vi "fittedresultdisplay.vi"(9 "x":dbl[](array[numeric]), 10 "num of gaussian peaks":i32, 11 "best fit parameters":dbl[](array[numeric])) -> (2 "resulting formula string":string, 3 "all gaussian points":T1(array[cluster]))   [LabVIEW 2020]
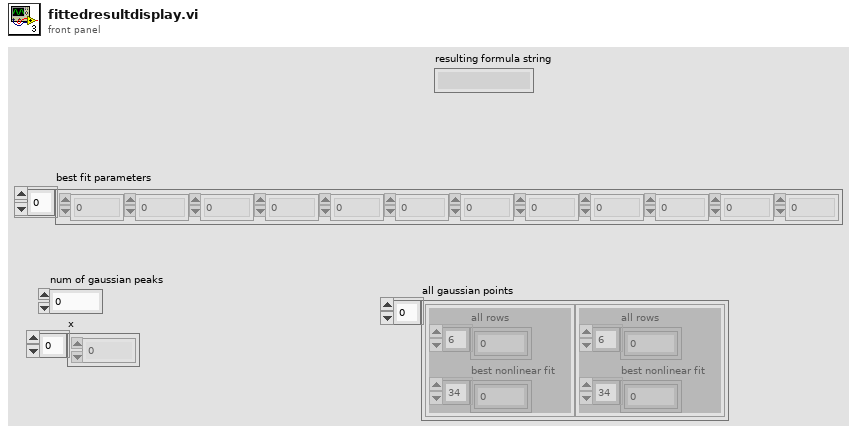
[diagram p1: front panel]
types:
  T1 = cluster{"all rows":dbl[], "best nonlinear fit":dbl[]}[]
  T2 = cluster{"all rows":dbl[], "best nonlinear fit":dbl[]}
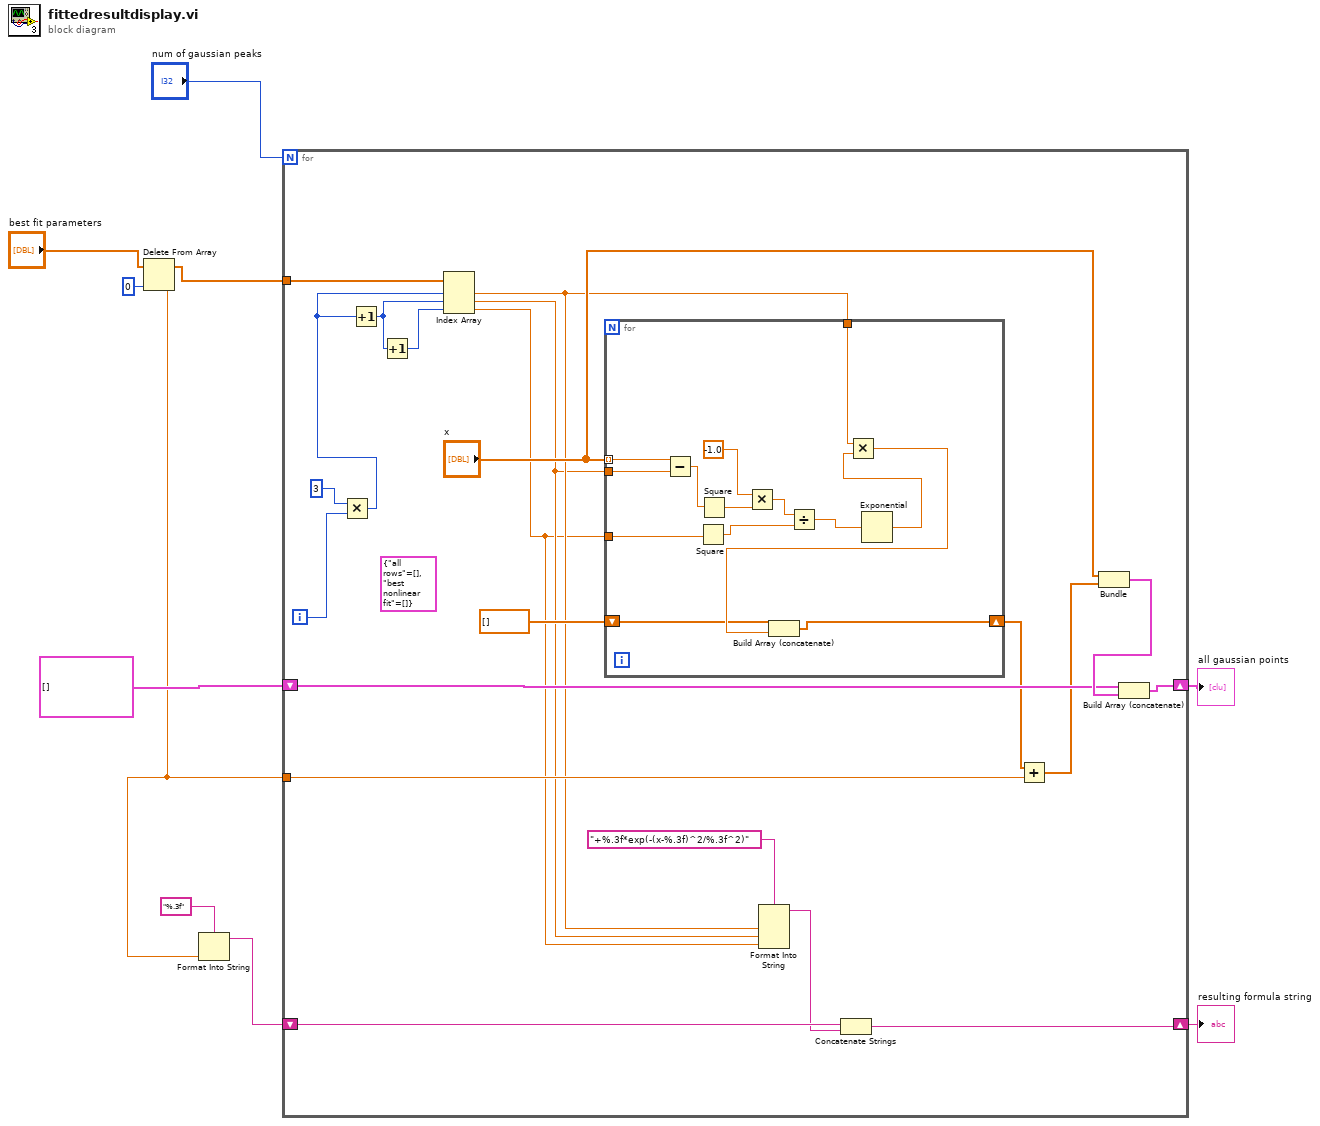
[diagram p0: block diagram]
diagram:
  n1 = Delete From Array(array="best fit parameters", index=0) -> (deleted portion=w3:dbl, array with subset deleted=w5:dbl[])  [unwired: 1 in]
  n2 = Format Into String(format string="%.3f", w3) -> (resulting string=w2:string)  [unwired: 2 in, 1 out]
  n3 = for {
    N: "num of gaussian peaks" -> [_]
    tunnel: w5 -> [w31]
    shift-right: [w21] -> w8
    shift-left: T1 [] ("appended array") -> [w22]
    tunnel: w3 -> [w18]
    shift-right: [w11] -> w1
    shift-left: w2 -> [w13]
    i -> [w30]
    (unwired) T2 {"all rows"=[], "best nonlinear fit"=[]}
    n4 = Multiply(x=3, y=w30) -> (x*y=w28:i32)
    n5 = Increment(x=w28) -> (x+1=w27:i32)
    n6 = Increment(x=w27) -> (x+1=w26:i32)
    n7 = Index Array(array=w31, index #1=w28, index #2=w27, index #3=w26) -> (element #1=w16:dbl, element #2=w15:dbl, element #3=w14:dbl)
    n8 = for {
      tunnel: "x" -> [w45] mode=indexing
      tunnel: w15 -> [w44]
      tunnel: w16 -> [w42]
      tunnel: w14 -> [w41]
      shift-right: [w32] -> w20
      shift-left: dbl[] [] ("y") -> [w33]
      n9 = Subtract(x=w45, y=w44) -> (x-y=w43:dbl)
      n10 = Square(x=w41) -> (x^2=w37:dbl)
      n11 = Square(x=w43) -> (x^2=w39:dbl)
      n12 = Multiply(x=-1.0, y=w39) -> (x*y=w38:dbl)
      n13 = Divide(x=w38, y=w37) -> (x/y=w36:dbl)
      n14 = Exponential(1:w36) -> (0:w35:dbl)
      n15 = Multiply(x=w42, y=w35) -> (x*y=w34:dbl)
      n16 = Build Array (concatenate)(w33, w34) -> (w32:dbl[])
    }
    n17 = Format Into String(format string="+%.3f*exp(-(x-%.3f)^2/%.3f^2)", w16, w15, w14) -> (resulting string=w12:string)  [unwired: 2 in, 1 out]
    n18 = Concatenate Strings(w13, w12) -> (w11:string)
    n19 = Add(x=w20, y=w18) -> (x+y=w19:dbl[])
    n20 = Bundle("x"="x", w19) -> (w23:cluster{"x":dbl[], dbl[]})  [unwired: 1 in]
    n21 = Build Array (concatenate)(w22, w23) -> (w21:cluster{"x":dbl[], "best nonlinear fit":dbl[]}[])
  }
  "all gaussian points" <- w8
  "resulting formula string" <- w1
